vi "Cluster to JSON.vi"() -> ()   [LabVIEW 2018, in "LV-Julia_ZMQ-Roundtrip_lib.lvlib"]
uses:
  LV-Julia_ZMQ-Roundtrip_lib.lvlib
panel:
  in  "str_arg":string
  in  "fun_name":string
  out "JSON string":string
  out "error out":errorcluster
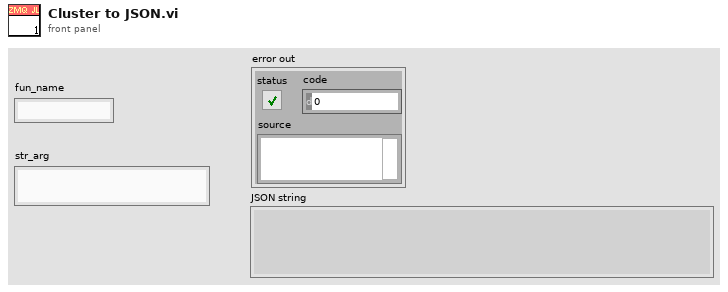
[diagram p1: front panel]
types:
  T1 = cluster{"fun_name":string, "str_arg":string, "Byte_array":u8[]}
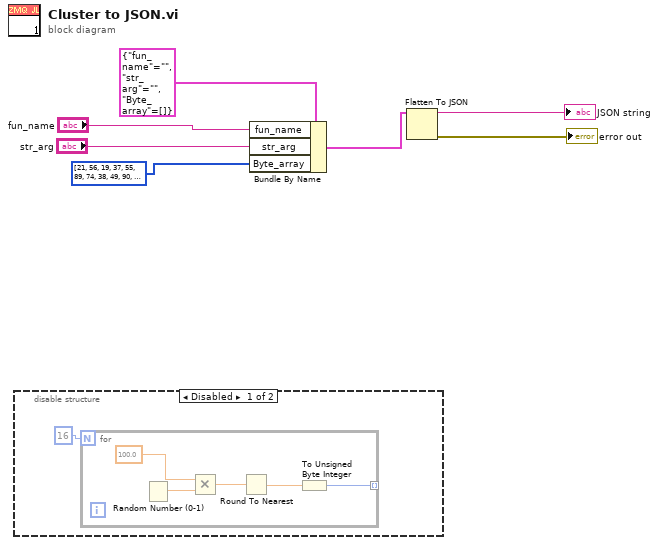
[diagram p0: block diagram]
diagram:
  n1 = disable-structure shown="Disabled" {
    frame Disabled {
      n2 = for {
        N: 16 -> [_]
        tunnel: [w9] -> _ mode=indexing
        n3 = Random Number (0-1)() -> (number: 0 to 1=w13:dbl)
        n4 = Multiply(x=100.0, y=w13) -> (x*y=w12:dbl)
        n5 = Round To Nearest(number=w12) -> (nearest integer value=w10:dbl)
        n6 = To Unsigned Byte Integer(number=w10) -> (unsigned 8bit integer=w9:u8)
      }
    }
    frame Enabled {
    }
  }
  n7 = Bundle By Name(cluster=T1 {"fun_name"="", "str_arg"="", "Byte_array"=[]} ("fun_cluster"), "fun_name"="fun_name", "str_arg"="str_arg", "Byte_array"=u8[] [21, 56, 19, 37, 55, 89, 74, 38, 49, 90, 2, 10, 96, 88, 14, 76] ("Array")) -> (w4:T1)
  n8 = Flatten To JSON(anything=w4) -> (JSON string=→"JSON string":string, 11:→"error out":errorcluster)  [unwired: 2 in]
